vi "Set Task Inactive.vi"(8 "error in (no error)":errorcluster, 9 "Task":string, 10 "Project":string, 11 "Projects in":refnum<class "Projects.lvclass">) -> (0 "error out":errorcluster, 3 "Projects out":refnum<class "Projects.lvclass">)   [LabVIEW 2020, in "Projects.lvclass"]
uses:
  Projects.lvclass
  Projects.lvclass/Projects.ctl
  <vilib>/Utility/miscctls.llb/LVMapReplaceAction.ctl
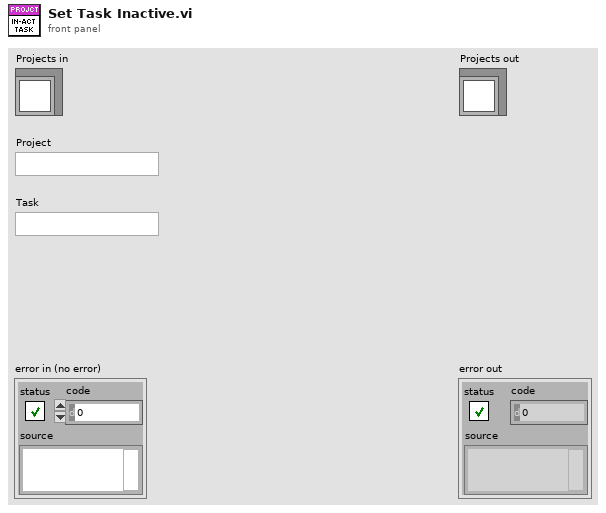
[diagram p1: front panel]
types:
  T1 = typedef "LVMapReplaceAction.ctl" = enum32{"Modify Entry only if found", "Add or Modify Entry", "Delete Entry"}
  T2 = typedef "Project Info.ctl" = cluster{"Project Active?":bool, "Tasks":set{string}, "Task Active":map{string, bool}}
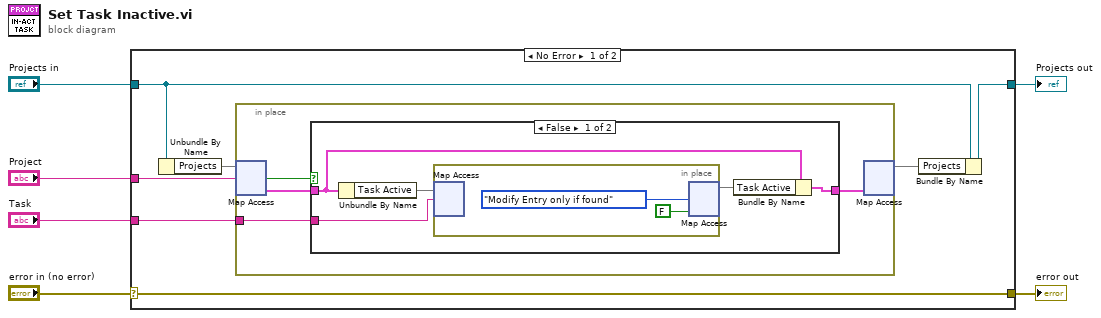
[diagram p0: block diagram]
diagram:
  n1 = case shown="No Error" "error in (no error)" {
    selector: "error in (no error)" -> [w13 w27]
    tunnel: [w13 w27] -> w5
    tunnel: [w8 w26] -> w3
    tunnel: "Projects in" -> [w12 w26]
    tunnel: "Project" -> [w10 _]
    tunnel: "Task" -> [w9 _]
    frame No Error {
      n2 = Unbundle By Name(w12) -> ("Projects"=w11:map{string, T2})
      n3 = in-place {
        in-place-border: w9 -> [w15]
        n4 = in-place-map #1(w11, w10) -> (w16:T2, w17:bool)  [unwired: 1 in]
        n5 = case shown="False" w17 {
          tunnel: w16 -> [w20 w25]
          tunnel: w15 -> [w21 _]
          tunnel: [w18 w25] -> w14
          frame False {
            n6 = Unbundle By Name(w20) -> ("Task Active"=w22:map{string, bool})
            n7 = in-place {
              n8 = in-place-map #2(w22, w21) -> ()  [unwired: 1 in, 2 out]
              n9 = in-place-map #2(FALSE ("value"), LVMapReplaceAction."Modify Entry only if found" ("action")) -> (w19:map{string, bool})  [unwired: 2 out]
            }
            n10 = Bundle By Name(cluster=w20, "Task Active"=w19) -> (w18:T2)
          }
          frame True {
          }
        }
        n11 = in-place-map #1(w14) -> (w7:map{string, T2})  [unwired: 1 in, 2 out]
      }
      n12 = Bundle By Name(cluster=w12, "Projects"=w7) -> (w8:refnum<class "Projects.lvclass">)
    }
    frame Error {
    }
  }
  "error out" <- w5
  "Projects out" <- w3
